vi "#116_MAV_MSG_SCALED_IMU2_DECODE.vi"(11 "mavlink_payload":u8[](array[numeric])) -> (3 "SCALED_IMU2":T1)   [LabVIEW 2023]
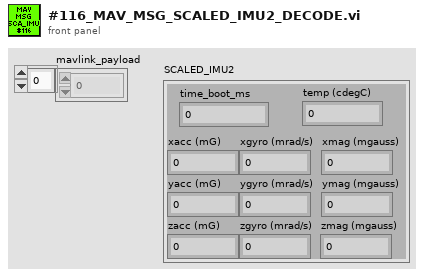
[diagram p1: front panel]
types:
  T1 = cluster{"time_boot_ms":u32, "xacc (mG)":i16, "yacc (mG)":i16, "zacc (mG)":i16, "xgyro (mrad/s)":i16, "ygyro (mrad/s)":i16, "zgyro (mrad/s)":i16, "xmag (mgauss)":i16, "ymag (mgauss)":i16, "zmag (mgauss)":i16, "temp (cdegC)":i16}
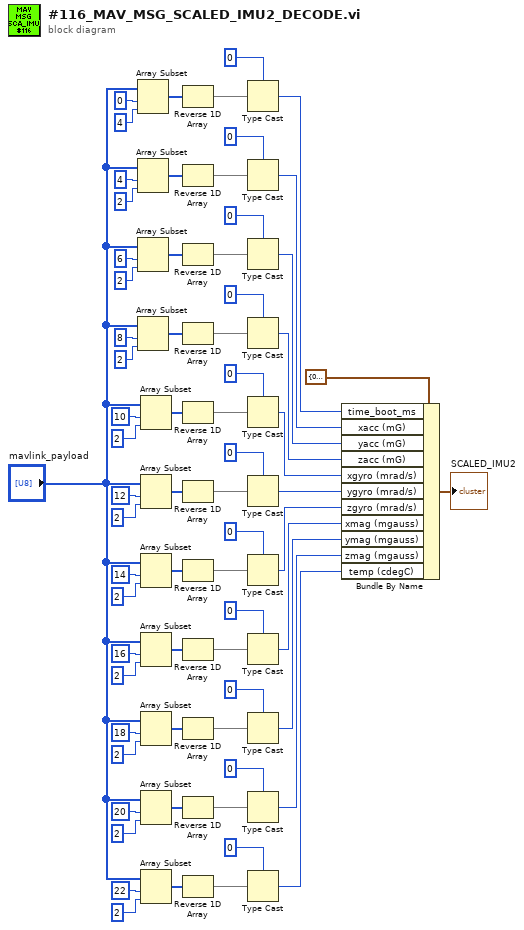
[diagram p0: block diagram]
diagram:
  n1 = Array Subset(array="mavlink_payload", index=0 ("Index"), length=4) -> (w68:u8[])
  n2 = Array Subset(array="mavlink_payload", index=4 ("Index"), length=2) -> (w60:u8[])
  n3 = Array Subset(array="mavlink_payload", index=6 ("Index"), length=2) -> (w54:u8[])
  n4 = Array Subset(array="mavlink_payload", index=8 ("Index"), length=2) -> (w48:u8[])
  n5 = Array Subset(array="mavlink_payload", index=10 ("Index"), length=2) -> (w42:u8[])
  n6 = Array Subset(array="mavlink_payload", index=12 ("Index"), length=2) -> (w36:u8[])
  n7 = Array Subset(array="mavlink_payload", index=14 ("Index"), length=2) -> (w30:u8[])
  n8 = Array Subset(array="mavlink_payload", index=16 ("Index"), length=2) -> (w24:u8[])
  n9 = Array Subset(array="mavlink_payload", index=18 ("Index"), length=2) -> (w18:u8[])
  n10 = Array Subset(array="mavlink_payload", index=20 ("Index"), length=2) -> (w12:u8[])
  n11 = Array Subset(array="mavlink_payload", index=22 ("Index"), length=2) -> (w6:u8[])
  n12 = Reverse 1D Array(array=w68) -> (reversed array=w67:u8[])
  n13 = Reverse 1D Array(array=w60) -> (reversed array=w59:u8[])
  n14 = Reverse 1D Array(array=w54) -> (reversed array=w53:u8[])
  n15 = Reverse 1D Array(array=w48) -> (reversed array=w47:u8[])
  n16 = Reverse 1D Array(array=w42) -> (reversed array=w41:u8[])
  n17 = Reverse 1D Array(array=w36) -> (reversed array=w35:u8[])
  n18 = Reverse 1D Array(array=w30) -> (reversed array=w29:u8[])
  n19 = Reverse 1D Array(array=w24) -> (reversed array=w23:u8[])
  n20 = Reverse 1D Array(array=w18) -> (reversed array=w17:u8[])
  n21 = Reverse 1D Array(array=w12) -> (reversed array=w11:u8[])
  n22 = Reverse 1D Array(array=w6) -> (reversed array=w5:u8[])
  n23 = Type Cast(type=u32 0 ("Index"), x=w67) -> (*(type *) &x=w62:u32)
  n24 = Type Cast(type=i16 0 ("Index"), x=w59) -> (*(type *) &x=w56:i16)
  n25 = Type Cast(type=i16 0 ("Index"), x=w53) -> (*(type *) &x=w50:i16)
  n26 = Type Cast(type=i16 0 ("Index"), x=w47) -> (*(type *) &x=w44:i16)
  n27 = Type Cast(type=i16 0 ("Index"), x=w41) -> (*(type *) &x=w38:i16)
  n28 = Type Cast(type=i16 0 ("Index"), x=w35) -> (*(type *) &x=w32:i16)
  n29 = Type Cast(type=i16 0 ("Index"), x=w29) -> (*(type *) &x=w26:i16)
  n30 = Type Cast(type=i16 0 ("Index"), x=w23) -> (*(type *) &x=w20:i16)
  n31 = Type Cast(type=i16 0 ("Index"), x=w17) -> (*(type *) &x=w14:i16)
  n32 = Type Cast(type=i16 0 ("Index"), x=w11) -> (*(type *) &x=w8:i16)
  n33 = Type Cast(type=i16 0 ("Index"), x=w5) -> (*(type *) &x=w1:i16)
  n34 = Bundle By Name(cluster=T1 {"time_boot_ms"=0, "xacc (mG)"=0, "yacc (mG)"=0, "zacc (mG)"=0, "xgyro (mrad/s)"=0, "ygyro (mrad/s)"=0, "zgyro (mrad/s)"=0, "xmag (mgauss)"=0, "ymag (mgauss)"=0, "zmag (mgauss)"=0, "temp (cdegC)"=0} ("SCALED_IMU2"), "time_boot_ms"=w62, "xacc (mG)"=w56, "yacc (mG)"=w50, "zacc (mG)"=w44, "xgyro (mrad/s)"=w38, "ygyro (mrad/s)"=w32, "zgyro (mrad/s)"=w26, "xmag (mgauss)"=w20, "ymag (mgauss)"=w14, "zmag (mgauss)"=w8, "temp (cdegC)"=w1) -> (→"SCALED_IMU2":T1)
